vi "get_image_name.vi"(11 "path":path) -> (3 "image_name":string)   [LabVIEW 2021]
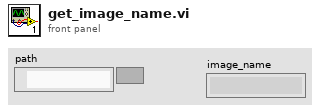
[diagram p1: front panel]
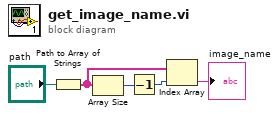
[diagram p0: block diagram]
diagram:
  n1 = Path to Array of Strings(0:"path") -> (2:w5:string[])  [unwired: 1 out]
  n2 = Array Size(array=w5) -> (size(s)=w4:i32)
  n3 = Decrement(x=w4) -> (x-1=w3:i32)
  n4 = Index Array(array=w5, index=w3) -> (element=→"image_name":string)
